vi "Alarms Set Event Response.vi"(8 "error in (no error)":errorcluster, 9 "Alarms":T1, 10 "Alarm Event":T3(ring), 11 "Alarms in":refnum<class "HK Alarms.lvclass">) -> (0 "error out":errorcluster, 3 "Alarms out":refnum<class "HK Alarms.lvclass">)   [LabVIEW 2019, in "HK Alarms.lvclass"]
uses:
  HK Alarms/HK Alarms.lvclass
  HK Channel Settings Alarms.ctl
  HK Alarm enum Action.ctl
  HK Alarms/HK Alarms.lvclass/HK Alarms.ctl
  HK Item/HK Item.lvclass
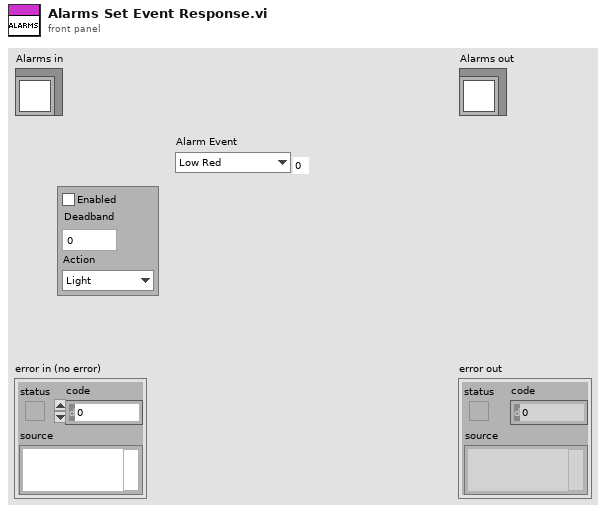
[diagram p1: front panel]
types:
  T1 = typedef "HK Item.lvclass/HK Channel Settings Alarms.ctl" = cluster{"Enabled":bool, "Deadband":i32, "Action":T2}
  T2 = typedef "HK Item.lvclass/HK Alarm enum Action.ctl" = enum16{"Light", "Message", "Safe"}
  T3 = enum16{"Low Red", "Low Yellow", "High Yellow", "High Red"}
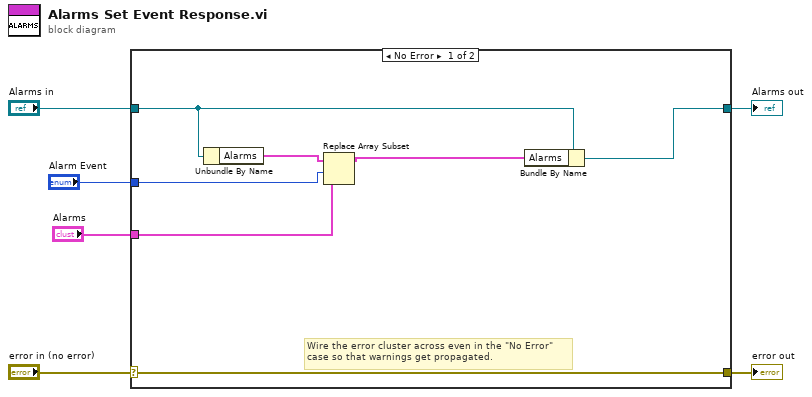
[diagram p0: block diagram]
diagram:
  n1 = case shown="No Error" "error in (no error)" {
    selector: "error in (no error)" -> [w13 w15]
    tunnel: [w13 w15] -> w5
    tunnel: [w8 w14] -> w3
    tunnel: "Alarms in" -> [w7 w14]
    tunnel: "Alarm Event" -> [w11 _]
    tunnel: "Alarms" -> [w10 _]
    frame No Error {
      # "Wire the error cluster across even in the \"No Error\"\ncase so that warnings get propagated."
      n2 = Unbundle By Name(w7) -> ("Alarms"=w12:T1[])
      n3 = Replace Array Subset(array=w12, new element=w10, index=w11) -> (w9:T1[])
      n4 = Bundle By Name(cluster=w7, "Alarms"=w9) -> (w8:refnum<class "HK Alarms.lvclass">)
    }
    frame Error {
    }
  }
  "error out" <- w5
  "Alarms out" <- w3
